vi "SVFA Unit Conversion.vi"   [LabVIEW 2017]
doc: "Converts between dB/linear, magnitude/magnitude^2, rms/peak/peak-peak, spectrum/spectral density, and dB ref1/dB ref2. Wire data to the <B>spectrum</B> input to determine the polymorphic instance to use or manually select the instance."
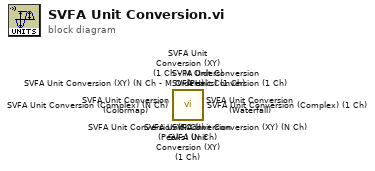
[diagram p0: block diagram]
diagram:
  n1 = call <vilib>:"SVFA Unit Conversion (Peaks) (N Ch).vi"() -> ()  [unwired: 16 in, 4 out]
  n2 = call <vilib>:"SVFA Unit Conversion (Peaks) (1 Ch).vi"() -> ()  [unwired: 16 in, 4 out]
  n3 = call <vilib>:"SVFA Unit Conversion (Colormap).vi"() -> ()  [unwired: 16 in, 4 out]
  n4 = call <vilib>:"SVFA Unit Conversion (Waterfall).vi"() -> ()  [unwired: 16 in, 4 out]
  n5 = call <vilib>:"SVFA Unit Conversion (XY) (N Ch - M Orders).vi"() -> ()  [unwired: 16 in, 4 out]
  n6 = call <vilib>:"SVFA Unit Conversion (XY) (1 Ch - M Orders).vi"() -> ()  [unwired: 16 in, 4 out]
  n7 = call <vilib>:"SVFA Unit Conversion (XY) (N Ch).vi"() -> ()  [unwired: 16 in, 4 out]
  n8 = call <vilib>:"SVFA Unit Conversion (XY) (1 Ch).vi"() -> ()  [unwired: 16 in, 4 out]
  n9 = call <vilib>:"SVFA Unit Conversion (Complex) (N Ch).vi"() -> ()  [unwired: 14 in, 6 out]
  n10 = call <vilib>:"SVFA Unit Conversion (Complex) (1 Ch).vi"() -> ()  [unwired: 14 in, 6 out]
  n11 = call <vilib>:"SVFA Unit Conversion (N Ch).vi"() -> ()  [unwired: 16 in, 4 out]
  n12 = call <vilib>:"SVFA Unit Conversion (1 Ch).vi"() -> ()  [unwired: 16 in, 4 out]
